vi "Set Gain Setting.vi"(0 "RedPitaya connection in":refnum<k5>, 3 "Gain Voltage":string(combo), 5 "error in":errorcluster, 8 "Channel":u16(ring)=1 items=["Channel 1"=1, "Channel 2"=2], 12 "timeout ms (2000)":i32=2000) -> (14 "RedPitaya connection out":refnum<k5>, 19 "error out":errorcluster)   [LabVIEW 2010, in "RedPitaya.lvlib"]
doc: "Set gain settings to HIGH or LOW. This gain is referring to jumper settings on Red Pitaya fast analog inputs."
uses:
  RedPitaya.lvlib
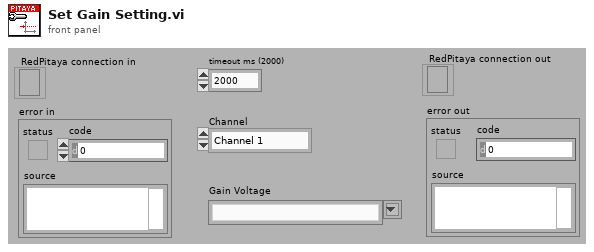
[diagram p1: front panel]
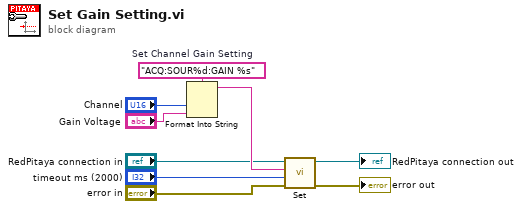
[diagram p0: block diagram]
diagram:
  w9 = "ACQ:SOUR%d:GAIN %s"  # Set Channel Gain Setting
  n1 = Format Into String(format string=w9, "Channel", "Gain Voltage") -> (resulting string=w7:string)  [unwired: 2 in, 1 out]
  n2 = call "Set.vi"("error in"="error in", "timeout ms (2000)"="timeout ms (2000)", "SCPI Message"=w7, "RedPitaya connection in"="RedPitaya connection in") -> ("error out"=→"error out":errorcluster, "RedPitaya connection out"=→"RedPitaya connection out":refnum<k5>)  [unwired: 5 in, 1 out]
